vi "SQLite Query - Create Table.vi"(8 "error in":errorcluster, 9 "Table Col SQL Data Types":string[](array[string]), 10 "Table Headers":string[](array[string]), 11 "Table Name":string) -> (0 "error out":errorcluster, 3 "SQLite Query":string)   [LabVIEW 2015, in "TableLogger_SQLite_Actor.lvlib" / "TableLogger_SQLite_Actor.lvclass"]
uses:
  TableLogger_SQLite_Actor.lvclass
panel:
  # "Connector Pane"
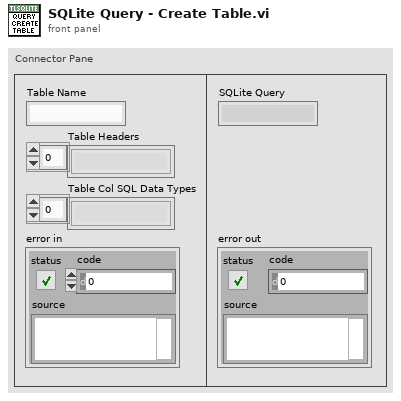
[diagram p1: front panel]
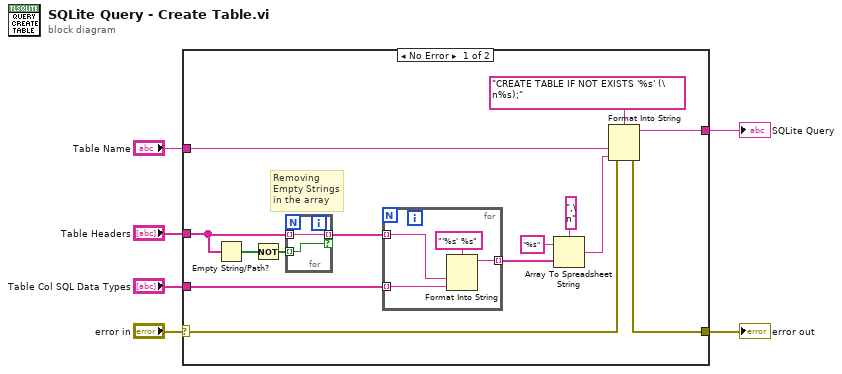
[diagram p0: block diagram]
diagram:
  n1 = case shown="No Error" "error in" {
    selector: "error in" -> [w8 w27]
    tunnel: "Table Col SQL Data Types" -> [w20 _]
    tunnel: [w19 _] -> w5
    tunnel: "Table Name" -> [w11 _]
    tunnel: "Table Headers" -> [w9 _]
    tunnel: [w7 w27] -> w1
    frame No Error {
      # "Removing Empty Strings in the array"
      n2 = Empty String/Path?(string/path=w9) -> (empty?=w15:bool[])
      n3 = Not(x=w15) -> (.not. x?=w16:bool[])
      n4 = for {
        tunnel: w16 -> [w21] mode=indexing
        tunnel: w9 -> [w22] mode=indexing
        tunnel: [w22] -> w17 mode=indexing if=w21
      }
      n5 = for {
        tunnel: [w24] -> w12 mode=indexing
        tunnel: w17 -> [w25] mode=indexing
        tunnel: w20 -> [w23] mode=indexing
        n6 = Format Into String(format string="'%s' %s", w25, w23) -> (resulting string=w24:string)  [unwired: 2 in, 1 out]
      }
      n7 = Array To Spreadsheet String(delimiter (Tab)=",\n", array=w12, 3:"%s" ("format string")) -> (spreadsheet string=w14:string)
      n8 = Format Into String(format string="CREATE TABLE IF NOT EXISTS '%s' (\n%s);" ("SQL"), error in=w8, w11, w14) -> (resulting string=w19:string, error out=w7:errorcluster)  [unwired: 1 in]
    }
    frame Error {
    }
  }
  "SQLite Query" <- w5
  "error out" <- w1
